vi "build database.vi"() -> ()   [LabVIEW 2014]
uses:
  <vilib>/Utility/file.llb/Read From Spreadsheet File (string).vi
  <vilib>/Utility/file.llb/Read From Spreadsheet File (I64).vi
panel:
  in  "Save combined file":path
  in  "Next Button":bool
  out "array w/ subset deleted":i64[][](array[numeric])
  out "output array":string[][](array[string])
  in  "Files to combine":cluster{"File in":path, "Flip":bool}[](array[cluster])
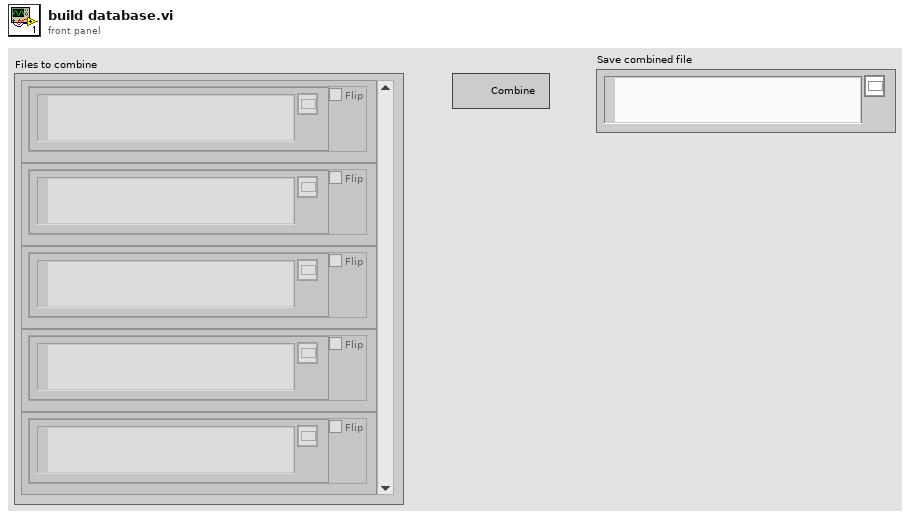
[diagram p1: front panel]
types:
  T1 = enum16{"open", "replace", "create", "open or create", "replace or create", "replace or create with confirmation"}
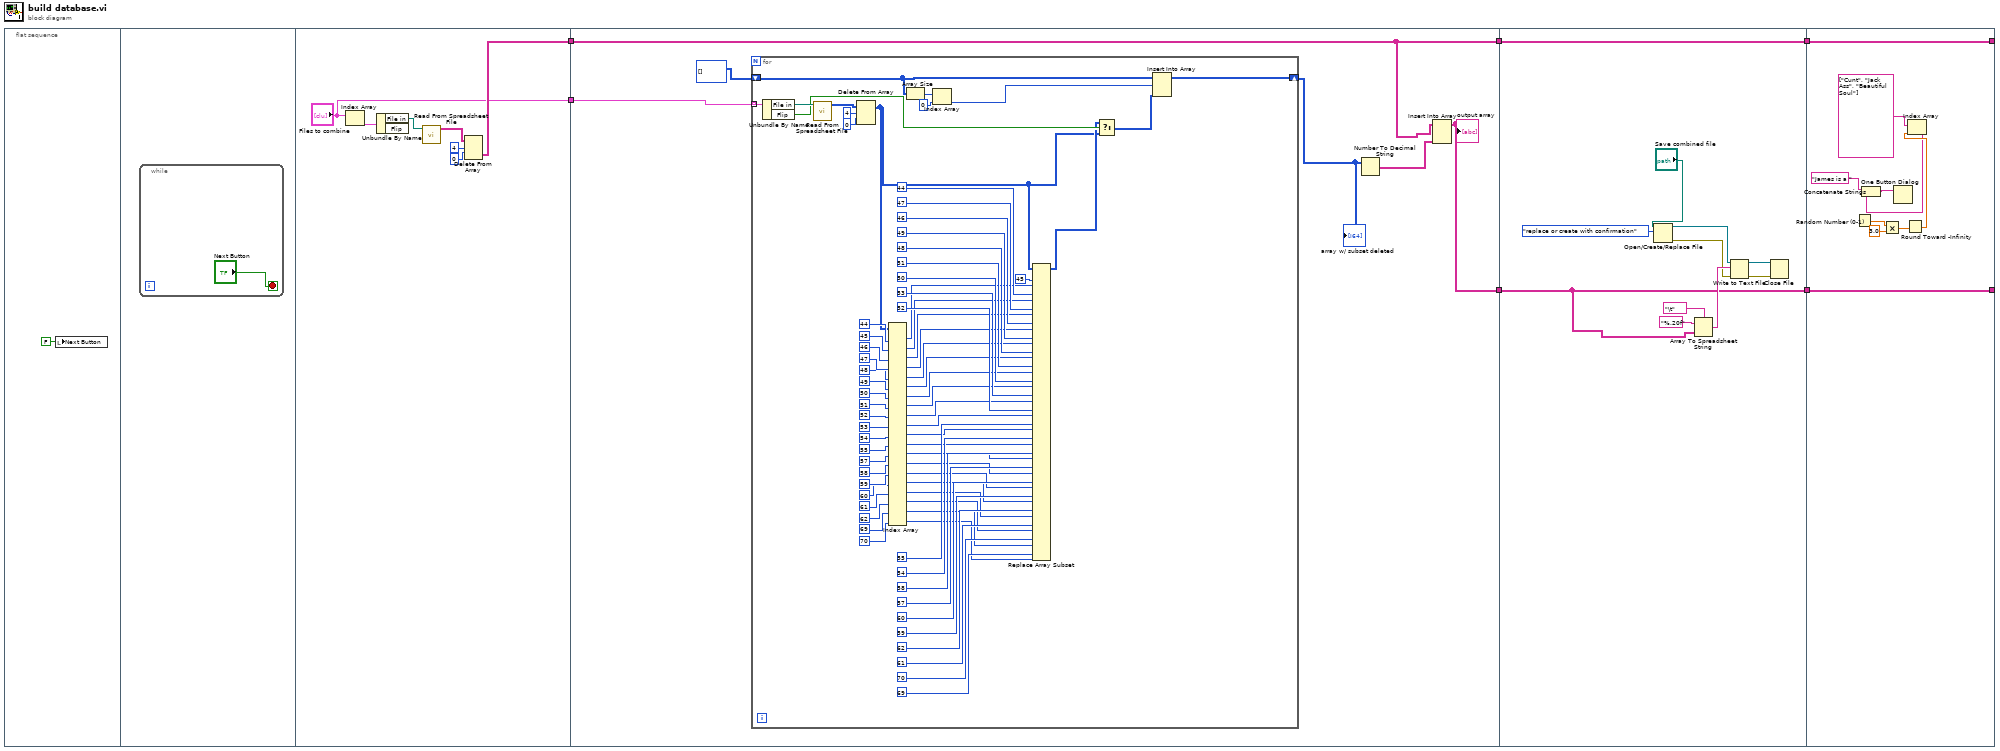
[diagram p0: block diagram]
diagram:
  n1 = flat-sequence {
    tunnel: [w10] -> w6
    tunnel: ["Files to combine"] -> w5
    tunnel: w6 -> [w18]
    tunnel: w5 -> [w19]
    tunnel: [w18] -> w4
    tunnel: [w16] -> w3
    tunnel: w4 -> [w106]
    tunnel: w3 -> [w96]
    tunnel: [w106] -> w2
    tunnel: [w96] -> w1
    tunnel: [w115] -> _
    tunnel: [w116] -> _
    tunnel: w2 -> [w116]
    tunnel: w1 -> [w115]
    frame #0 {
      n2 = local write "Next Button"(FALSE ("Next Button")) -> ()
    }
    frame #1 {
      n3 = while {
        stop <- "Next Button" stop-if-true
      }
    }
    frame #2 {
      n4 = Index Array(array="Files to combine") -> (element=w15:cluster{"File in":path, "Flip":bool})  [unwired: 1 in]
      n5 = Unbundle By Name(w15) -> ("File in"=w14:path)  [unwired: 1 out]
      n6 = call-poly <vilib>:"Read From Spreadsheet File.vi"("file path (dialog if empty)"=w14) -> ("all rows"=w11:string[][])  [unwired: 6 in, 4 out]
      n7 = Delete From Array(array=w11, length=4, index (row)=0) -> (deleted portion=w10:string[][])  [unwired: 1 in, 1 out]
    }
    frame #3 {
      n8 = for {
        tunnel: w19 -> [w95] mode=indexing
        shift-right: [w88] -> w20
        shift-left: i64[][] [] ("array w/ subset deleted") -> [w90]
        n9 = Unbundle By Name(w95) -> ("File in"=w91:path, "Flip"=w25:bool)
        n10 = call-poly <vilib>:"Read From Spreadsheet File.vi"("file path (dialog if empty)"=w91) -> ("all rows"=w92:i64[][])  [unwired: 6 in, 4 out]
        n11 = Delete From Array(array=w92, length=4, index (row)=0) -> (array with subset deleted=w23:i64[][])  [unwired: 1 in, 1 out]
        n12 = Index Array(array=w23, index (col) #1=44 ("disabled index (col)"), index (col) #2=45 ("disabled index (col)"), index (col) #3=46 ("disabled index (col)"), index (col) #4=47 ("disabled index (col)"), index (col) #5=48 ("disabled index (col)"), index (col) #6=49 ("disabled index (col)"), index (col) #7=50 ("disabled index (col)"), index (col) #8=51 ("disabled index (col)"), index (col) #9=52 ("disabled index (col)"), index (col) #10=53 ("disabled index (col)"), index (col) #11=54 ("disabled index (col)"), index (col) #12=55 ("disabled index (col)"), index (col) #13=57 ("disabled index (col)"), index (col) #14=58 ("disabled index (col)"), index (col) #15=59 ("disabled index (col)"), index (col) #16=60 ("disabled index (col)"), index (col) #17=61 ("disabled index (col)"), index (col) #18=62 ("disabled index (col)"), index (col) #19=69 ("disabled index (col)"), index (col) #20=70 ("disabled index (col)")) -> (element #1=w45:i64[], element #2=w44:i64[], element #3=w43:i64[], element #4=w42:i64[], element #5=w41:i64[], element #6=w40:i64[], element #7=w39:i64[], element #8=w38:i64[], element #9=w37:i64[], element #10=w36:i64[], element #11=w35:i64[], element #12=w34:i64[], element #13=w33:i64[], element #14=w32:i64[], element #15=w31:i64[], element #16=w30:i64[], element #17=w29:i64[], element #18=w28:i64[], element #19=w27:i64[], element #20=w26:i64[])  [unwired: 20 in]
        n13 = Array Size(array=w90) -> (size(s)=w89:i32[])
        n14 = Index Array(array=w89, index=0) -> (element=w87:i32)
        n15 = Replace Array Subset(array=w23, new element #1=w45, index (col) #1=45 ("disabled index (col)"), new element #2=w44, index (col) #2=44 ("disabled index (col)"), new element #3=w43, index (col) #3=47 ("disabled index (col)"), new element #4=w42, index (col) #4=46 ("disabled index (col)"), new element #5=w41, index (col) #5=49 ("disabled index (col)"), new element #6=w40, index (col) #6=48 ("disabled index (col)"), new element #7=w39, index (col) #7=51 ("disabled index (col)"), new element #8=w38, index (col) #8=50 ("disabled index (col)"), new element #9=w37, index (col) #9=53 ("disabled index (col)"), new element #10=w36, index (col) #10=52 ("disabled index (col)"), new element #11=w35, index (col) #11=55 ("disabled index (col)"), new element #12=w34, index (col) #12=54 ("disabled index (col)"), new element #13=w33, index (col) #13=58 ("disabled index (col)"), new element #14=w32, index (col) #14=57 ("disabled index (col)"), new element #15=w31, index (col) #15=60 ("disabled index (col)"), new element #16=w30, index (col) #16=59 ("disabled index (col)"), new element #17=w29, index (col) #17=62 ("disabled index (col)"), new element #18=w28, index (col) #18=61 ("disabled index (col)"), new element #19=w27, index (col) #19=70 ("disabled index (col)"), new element #20=w26, index (col) #20=69 ("disabled index (col)")) -> (w24:i64[][])  [unwired: 20 in]
        n16 = Select(t=w24, s=w25, f=w23) -> (s? t:f=w22:i64[][])
        n17 = Insert Into Array(array=w90, index (row)=w87, new element=w22) -> (w88:i64[][])  [unwired: 1 in]
      }
      "array w/ subset deleted" <- w20
      n18 = Number To Decimal String(number=w20) -> (decimal integer string=w17:string[][])  [unwired: 1 in]
      n19 = Insert Into Array(array=w18, new element=w17) -> (w16:string[][])  [unwired: 2 in]
      "output array" <- w16
    }
    frame #4 {
      n20 = Open/Create/Replace File(file path (use dialog)="Save combined file", operation (0:open)=T1."replace or create with confirmation") -> (refnum out=w100:refnum<file>, error out=w99:errorcluster)  [unwired: 4 in, 1 out]
      n21 = Array To Spreadsheet String(delimiter (Tab)="\t" ("delimiter (\\t)"), array=w96, 3:"%.20f" ("format (%.3f)")) -> (spreadsheet string=w104:string)
      n22 = Write to Text File(file (use dialog)=w100, text=w104, error in=w99) -> (refnum out=w98:refnum<file>, error out=w97:errorcluster)  [unwired: 1 in, 1 out]
      n23 = Close File(refnum=w98, error in=w97) -> ()  [unwired: 2 out]
    }
    frame #5 {
      n24 = Random Number (0-1)() -> (number: 0 to 1=w112:dbl)
      n25 = Multiply(x=w112, y=3.0) -> (x*y=w114:dbl)
      n26 = Round Toward -Infinity(1:w114) -> (0:w110:dbl)
      n27 = Index Array(array=string[] ["Cunt", "Jack Ass", "Beautiful Soul"], index=w110) -> (element=w108:string)
      n28 = Concatenate Strings("James is a " ("message"), w108) -> (w107:string)
      n29 = One Button Dialog(message=w107) -> ()  [unwired: 1 in, 1 out]
    }
  }
